vi "Read Tags.vi"(11 "Series in":refnum<class "Series.lvclass">) -> (2 "Tags":T1[](array[typedef]), 3 "Series out":refnum<class "Series.lvclass">)   [LabVIEW 2018, in "InfluxDB Client.lvlib" / "Series.lvclass"]
uses:
  Series.lvclass
  Controls/TagSet.ctl
  Series.lvclass/Series.ctl
  InfluxDB Client.lvlib
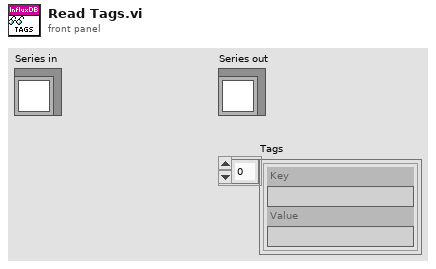
[diagram p1: front panel]
types:
  T1 = typedef "InfluxDB Client.lvlib/TagSet.ctl" = cluster{"Key":string, "Value":string}
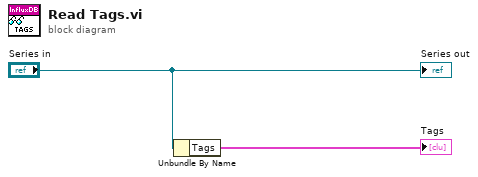
[diagram p0: block diagram]
diagram:
  n1 = Unbundle By Name("Series in") -> ("Tags"=→"Tags":T1[])
  "Series out" <- "Series in"
